vi "Query.vi"(2 "Condition":string, 3 "Error in":errorcluster, 4 "Table Name":string, 5 "Connection Name":string) -> (0 "Error out":errorcluster, 1 "data":string[][](array[string]))   [LabVIEW 2019, in "Database Lib.lvlib"]
uses:
  <vilib>/addons/database/Connection.llb/DB Tools Open Connec (String).vi
  <vilib>/addons/database/_DB Variant To Data/Database Variant To Data.xnode
  Database Lib.lvlib
  <vilib>/addons/database/NI_Database_API.lvlib
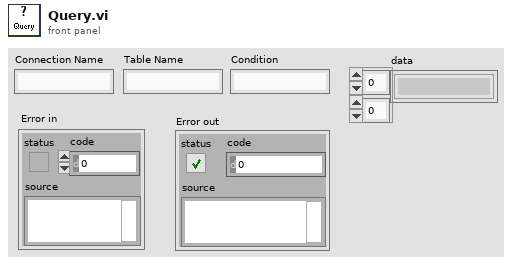
[diagram p1: front panel]
types:
  T1 = typedef "NI_Database_API.lvlib/Conn ObjectReference.ctl" = refnum<k1>
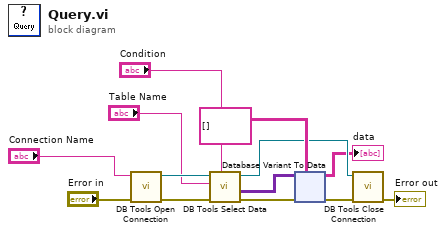
[diagram p0: block diagram]
diagram:
  n1 = call-poly <vilib>:"DB Tools Open Connection.vi"("error in (no error)"="Error in", "connection information"="Connection Name") -> ("error out"=w5:errorcluster, "connection reference"=w4:T1)  [unwired: 6 in]
  n2 = call <vilib>:"DB Tools Select Data.vi"("condition"="Condition", "error in (no error)"=w5, "table"="Table Name", "connection reference"=w4) -> ("error out"=w11:errorcluster, "data"=w12:variant[][], "connection reference out"=w6:T1)  [unwired: 2 in]
  n3 = xnode "Database Variant To Data"("database variant"=w12, "error in (no error)"=w11, "type"=string[][] []) -> ("data"=→"data":string[][], "error out"=w8:errorcluster)
  n4 = call <vilib>:"DB Tools Close Connection.vi"("error in (no error)"=w8, "connection reference"=w6) -> ("error out"=→"Error out":errorcluster)  [unwired: 5 in]
